vi "Sample_CoEIndexRead.vi"() -> ()   [LabVIEW 2022 SP3, in "EtherCAT_Library.lvlib"]
uses:
  EtherCAT_Library.lvlib
panel:
  out "Data":u8[](array[numeric])
  out "Entry name":string
  out "CoE Entry":T1
  in  "SubIndex":u8
  out "element":u16
  in  "index":i32
  out "Object description":T2 {"Index" format="%x"}
  out "Object name":string
  out "Device address 3":string
  in  "Device address":string
  in  "List type":T3(ring)
  out "List":u16[](array[numeric]) format="%x"
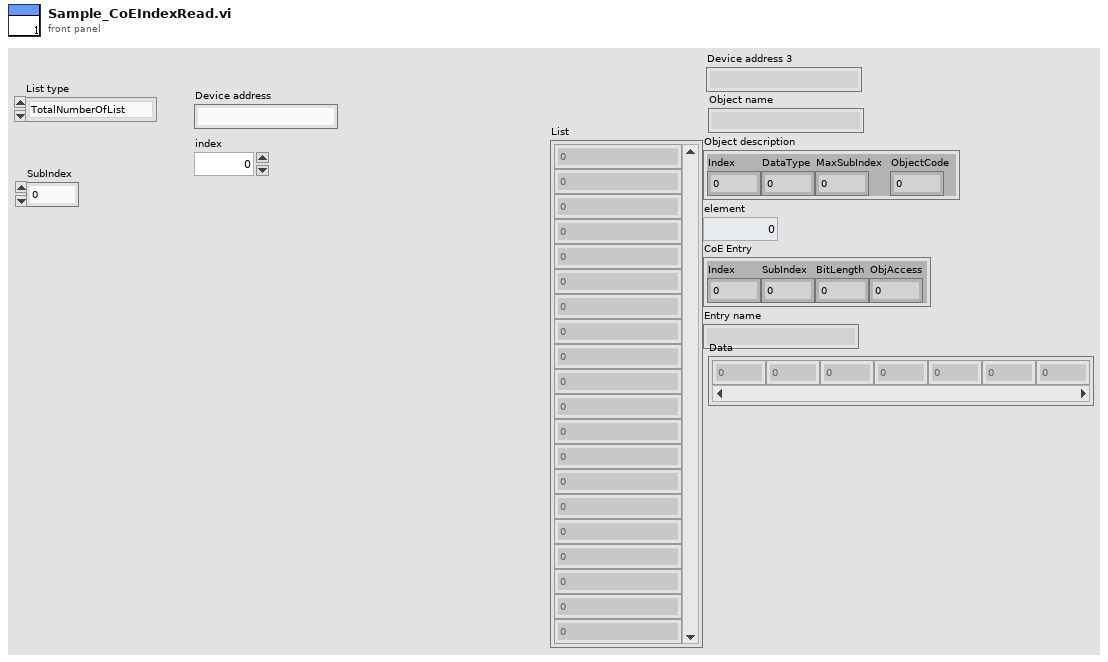
[diagram p1: front panel]
types:
  T1 = cluster{"Index":u16, "SubIndex":u8, "BitLength":u16, "ObjAccess":u16}
  T2 = cluster{"Index":u16, "DataType":u16, "MaxSubIndex":u8, "ObjectCode":u16}
  T3 = enum32{"TotalNumberOfList", "AllCoEObjects", "RxPDOs", "TxPDOs", "StoredForDevice", "StartUp"}
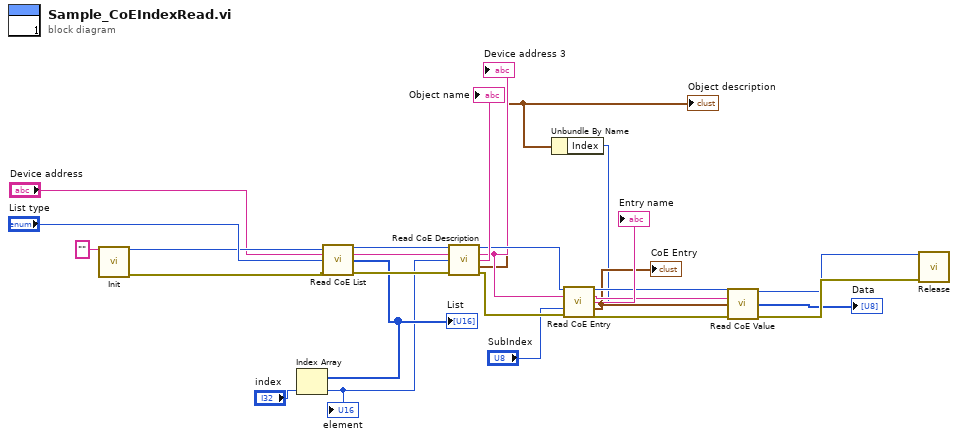
[diagram p0: block diagram]
diagram:
  n1 = call <userlib>:"Init.vi"("XMLDescription"="") -> ("Handle"=w25:u32, "error out"=w22:errorcluster)  [unwired: 10 in, 3 out]
  n2 = call <userlib>:"Read CoE List.vi"("Handle"=w25, "Device address"="Device address", "List type"="List type", "error in (no error)"=w22) -> ("Handle"=w21:u32, "Device address"=w19:string, "List"=w17:u16[], "error out"=w20:errorcluster)  [unwired: 8 in]
  "List" <- w17
  n3 = Index Array(array=w17, index="index") -> (element=w15:u16)
  "element" <- w15
  n4 = call <userlib>:"Read CoE Description.vi"("Handle"=w21, "Device address"=w19, "Index"=w15, "error in (no error)"=w20) -> ("Handle"=w14:u32, "Device address"=w12:string, "Object name"=→"Object name":string, "Object description"=w2:T2, "error out"=w13:errorcluster)  [unwired: 7 in]
  "Device address 3" <- w12
  "Object description" <- w2
  n5 = Unbundle By Name(w2) -> ("Index"=w1:u16)
  n6 = call <userlib>:"Read CoE Entry.vi"("Handle"=w14, "Device address"=w12, "Index"=w1, "SubIndex"="SubIndex", "error in (no error)"=w13) -> ("Handle"=w9:u32, "Device address"=w8:string, "Entry name"=→"Entry name":string, "CoE Entry"=w7:T1, "error out"=w6:errorcluster)  [unwired: 6 in]
  "CoE Entry" <- w7
  n7 = call <userlib>:"Read CoE Value.vi"("Handle"=w9, "Device address"=w8, "CoE entry"=w7, "error in (no error)"=w6) -> ("Handle"=w4:u32, "Data"=→"Data":u8[], "error out"=w5:errorcluster)  [unwired: 8 in, 1 out]
  n8 = call <userlib>:"Release.vi"("Handle"=w4, "error in (no error)"=w5) -> ()  [unwired: 13 in, 1 out]
